vi "Leading Edge Latch.vi"(1 "Input":bool) -> (0 "Output":bool)   [LabVIEW 2015]
doc: "This VI holds a true value one cycle after the false switches to true. In a real life button press this would hold true one cycle after the button is pressed and hold false for all other cases. Suggested implementation is a bump where after the bump the motor continues moving."
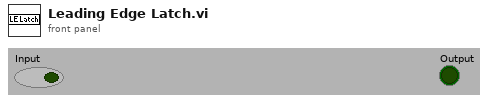
[diagram p1: front panel]
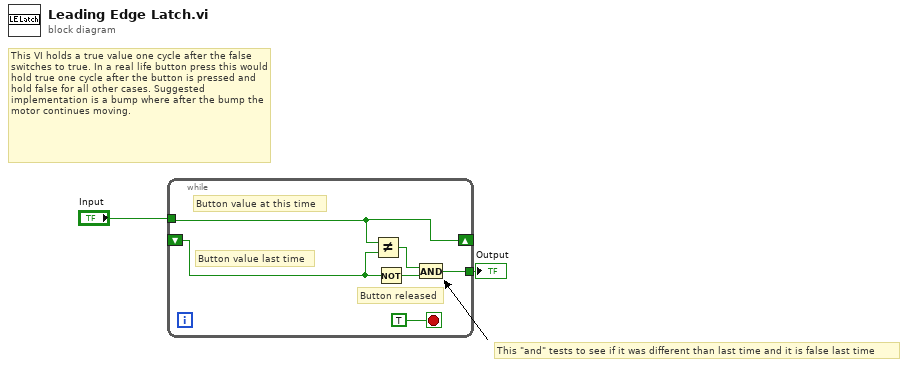
[diagram p0: block diagram]
diagram:
  # "This \"and\" tests to see if it was different than last time and it is false last time"
  # "This VI holds a true value one cycle after the false switches to true. In a real life button press this would hold true one cycle after the button is pressed and hold false for all other cases. Suggested implementation is a bump where after the bump the motor continues moving."
  n1 = while {
    tunnel: [w7] -> w1
    tunnel: "Input" -> [w6]
    shift-right: [w6] -> _
    shift-left: _ -> [w5]
    stop <- TRUE ("stop") stop-if-true
    # "Button released"
    # "Button value last time"
    # "Button value at this time"
    n2 = Not Equal?(x=w6, y=w5) -> (x != y?=w8:bool)
    n3 = Not(x=w5) -> (.not. x?=w3:bool)
    n4 = And(x=w8, y=w3) -> (x .and. y?=w7:bool)
  }
  "Output" <- w1
